vi "rec_manipMultiJumpDAQreplicates_v02.vi"(0 "AI task in":refnum<k21>, 1 "number of samples":i32=-1, 2 "Jump Position Array":T1(array[ring]), 3 "controls array in":refnum<vi>[](array[refnum]), 4 "AO task in":refnum<k21>, 5 "error in":errorcluster, 6 "Start Position":T2(ring), 7 "Delay":dbl, 8 "Use Current Position for Start Pos?":bool, 9 "Duration (s)":dbl, 11 "Position Dwell Time (s)":dbl[](array[numeric]), 12 "common cluster":T3) -> (14 "AI task out":refnum<k21>, 15 "data out (pA or mV)":waveform(dbl)(graph), 17 "control array out":refnum<vi>[](array[refnum]), 18 "AO task out":refnum<k21>, 19 "error out":errorcluster)   [LabVIEW 2019]
uses:
  multipatch/controls/multipatch_common_controls_v4.ctl
  machine_vision/controls/transform_cluster_actuator.ctl
  machine_vision/coordinate model vis/transform_properties_actuators.ctl
  pipette cleaning/pressure box/cleaning_soft/controls/actuator_cluster.ctl
  pipette cleaning/pressure box/cleaning_soft/controls/actuator_type.ctl
  pipette cleaning/pressure box/cleaning_soft/controls/pressure_box_control.ctl
  pipette cleaning/pressure box/cleaning_soft/controls/pressure_box_type.ctl
  controls/NH_method.ctl
  <vilib>/DAQmx/read.llb/DAQmx Read (Analog Wfm 1Chan NSamp).vi
  <vilib>/DAQmx/miscellaneous.llb/DAQmx Fill In Error Info.vi
  <resource>/objmgr/daqmx.rc
panel:
  out "AvailSampPerChan":u32
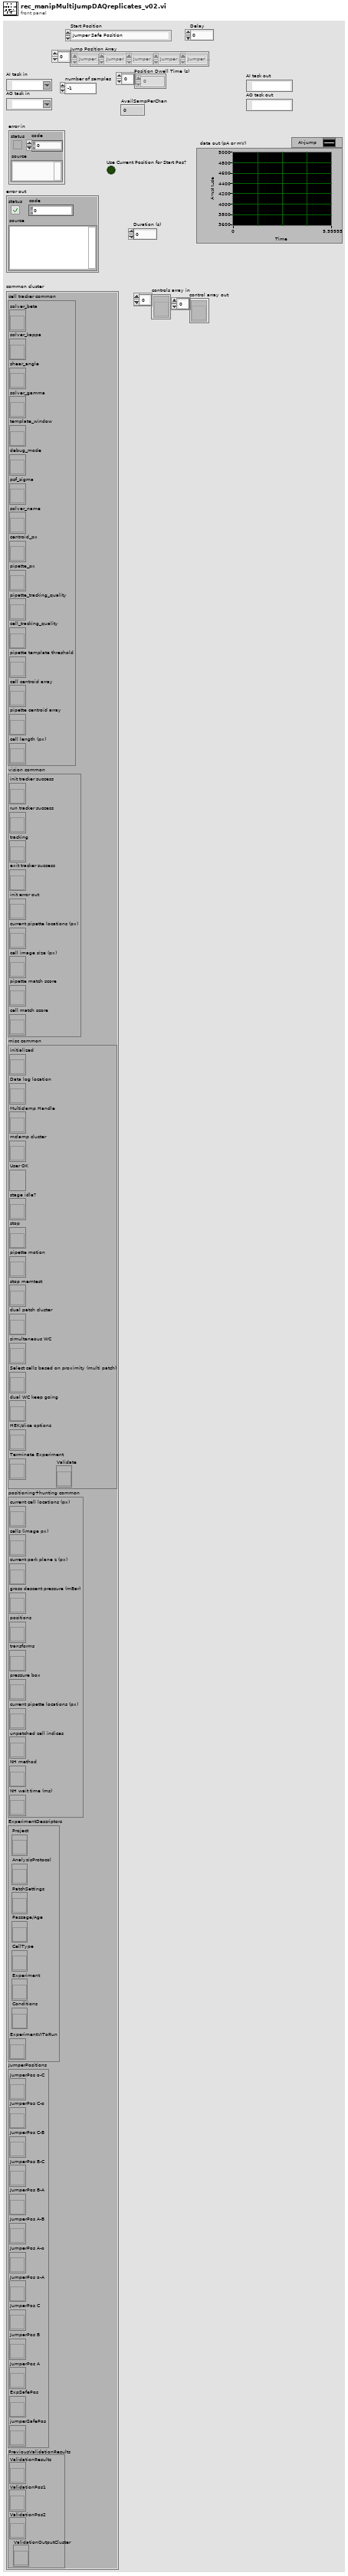
[diagram p1: front panel]
types:
  T1 = enum16{"Jumper Safe Position", "Experiment Safe Position", "Jumper Position A", "Jumper Position B", "Jumper Position C", "Jumper Position o-A", "Jumper Position A-o", "Jumper Position A-B", "Jumper Position B-A", "Jumper Position B-C", "Jumper Position C-B", "Jumper Position C-o", "Jumper Position o-C"}[]
  T2 = enum16{"Jumper Safe Position", "Experiment Safe Position", "Jumper Position A", "Jumper Position B", "Jumper Position C", "Jumper Position o-A", "Jumper Position A-o", "Jumper Position A-B", "Jumper Position B-A", "Jumper Position B-C", "Jumper Position C-B", "Jumper Position C-o", "Jumper Position o-C"}
  T3 = typedef "multipatch_common_controls_v4.ctl" = cluster{"cell tracker common":cluster{"solver_beta":refnum<vi>, "solver_kappa":refnum<vi>, "shear_angle":refnum<vi>, "solver_gamma":refnum<vi>, "template_window":refnum<vi>, "debug_mode":refnum<vi>, "psf_sigma":refnum<vi>, "solver_name":refnum<vi>, "centroid_px":refnum<vi>, "pipette_px":refnum<vi>, "pipette_tracking_quality":refnum<vi>, "cell_tracking_quality":refnum<vi>, "pipette template threshold":refnum<vi>, "cell centroid array":refnum<vi>, "pipette centroid array":refnum<vi>, "cell length (px)":refnum<vi>}, "vision common":cluster{"init tracker success":refnum<vi>, "run tracker success":refnum<vi>, "tracking":refnum<vi>, "exit tracker success":refnum<vi>, "init error out":refnum<vi>, "current pipette locations (px)":refnum<vi>, "cell image size (px)":refnum<vi>, "pipette match score":refnum<vi>, "cell match score":refnum<vi>}, "misc common":cluster{"initialized":refnum<vi>, "Data log location":refnum<vi>, "Multiclamp Handle":refnum<vi>, "mclamp cluster":refnum<vi>, "User OK":refnum<vi>, "stage idle?":refnum<vi>, "stop":refnum<vi>, "pipette motion":refnum<vi>, "stop memtest":refnum<vi>, "dual patch cluster":refnum<vi>, "simultaneous WC":refnum<vi>, "Select cells based on proximity (multi patch)":refnum<vi>, "dual WC keep going":refnum<vi>, "HEK/slice options":refnum<vi>, "Terminate Experiment":refnum<vi>, "Validate":refnum<vi>}, "positioning+hunting common":cluster{"current cell locations (px)":refnum<vi>, "cells (image px)":refnum<vi>, "current park plane z (px)":refnum<vi>, "gross descent pressure (mBar)":refnum<vi>, "positions":refnum<vi>, "transforms":refnum<vi>, "pressure box":refnum<vi>, "current pipette locations (px)":refnum<vi>, "unpatched cell indices":refnum<vi>, "NH method":refnum<vi>, "NH wait time (ms)":refnum<vi>}, "ExperimentDescriptors":cluster{"Project":refnum<vi>, "AnalysisProtocol":refnum<vi>, "PatchSettings":refnum<vi>, "Passage/Age":refnum<vi>, "CellType":refnum<vi>, "Experiment":refnum<vi>, "Conditions":refnum<vi>, "ExperimentVIToRun":refnum<vi>}, "JumperPositions":cluster{"JumperPos o-C":refnum<vi>, "JumperPos C-o":refnum<vi>, "JumperPos C-B":refnum<vi>, "JumperPos B-C":refnum<vi>, "JumperPos B-A":refnum<vi>, "JumperPos A-B":refnum<vi>, "JumperPos A-o":refnum<vi>, "JumperPos o-A":refnum<vi>, "JumperPos C":refnum<vi>, "JumperPos B":refnum<vi>, "JumperPos A":refnum<vi>, "ExpSafePos":refnum<vi>, "jumperSafePos":refnum<vi>}, "PreviousValidationResults":cluster{"ValidationResults":refnum<vi>, "ValidationPos1":refnum<vi>, "ValidationPos2":refnum<vi>, "ValidationOutputCluster":refnum<vi>}}
  T4 = enum16{"manipulator 1", "manipulator 2", "manipulator 3", "manipulator 4"}
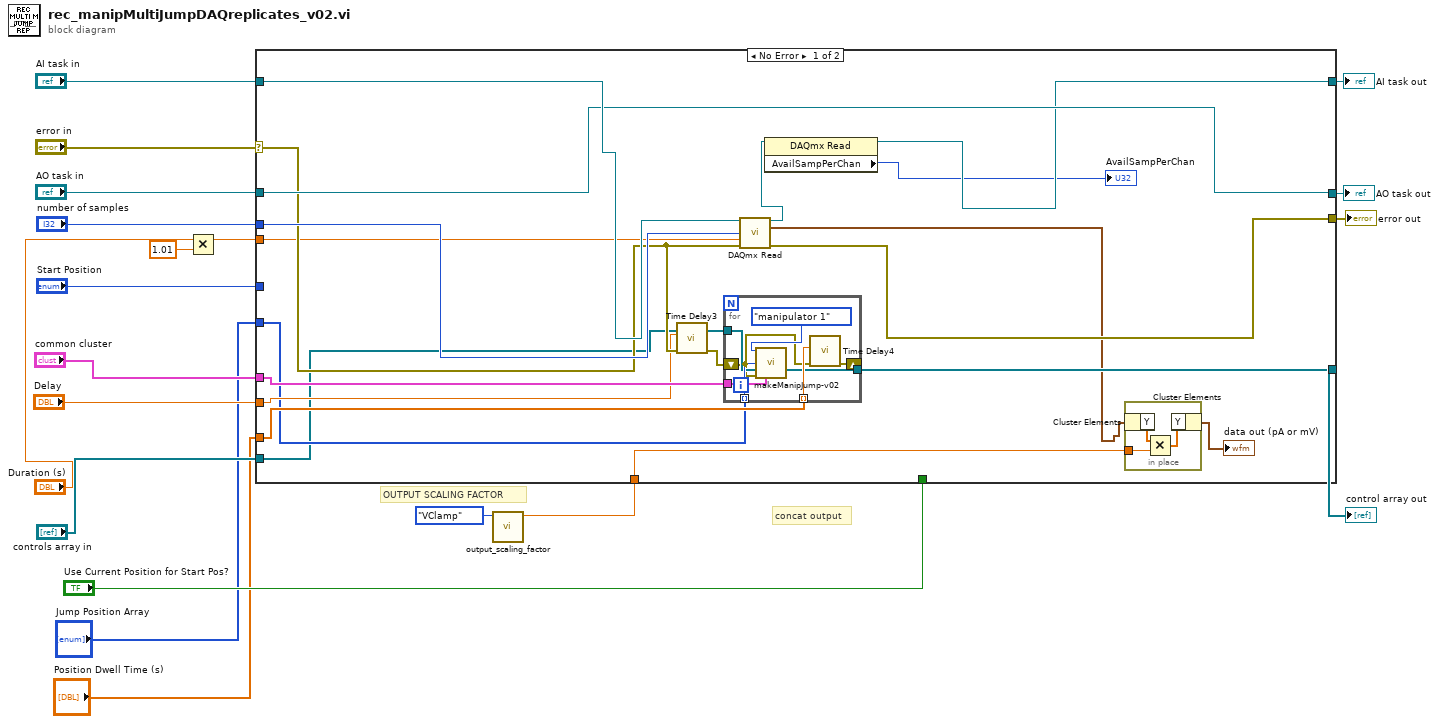
[diagram p0: block diagram]
diagram:
  # "concat output"
  # "OUTPUT SCALING FACTOR"
  n1 = Multiply(x="Duration (s)", y=1.01) -> (x*y=w5:dbl)
  n2 = call "output_scaling_factor.vi"("which clamp"=enum16{"VClamp", "IClamp"}."VClamp") -> ("output scaling factor"=w14:dbl)  [unwired: 10 in]
  n3 = case shown="No Error" "error in" {
    selector: "error in" -> [w34 w52]
    tunnel: "AI task in" -> [w38 w54]
    tunnel: "AO task in" -> [w36 w53]
    tunnel: [w36 w53] -> w17
    tunnel: [w27 w54] -> w16
    tunnel: [w37 w52] -> w15
    tunnel: w14 -> [w39 _]
    tunnel: "number of samples" -> [w35 _]
    tunnel: "common cluster" -> [w33 _]
    tunnel: "Delay" -> [w32 _]
    tunnel: "Position Dwell Time (s)" -> [w31 _]
    tunnel: "Start Position" -> [_ _]
    tunnel: "Jump Position Array" -> [w30 _]
    tunnel: "controls array in" -> [w29 w51]
    tunnel: [w28 w51] -> w7
    tunnel: w5 -> [w25 _]
    tunnel: "Use Current Position for Start Pos?" -> [_ _]
    frame No Error {
      n4 = call "Time Delay3"("error in (no error)"=w34, "Delay Time (s)"=w32) -> ("error out"=w23:errorcluster)  [unwired: 9 in]
      n5 = for {
        tunnel: w33 -> [w50]
        tunnel: w31 -> [w49] mode=indexing
        tunnel: w30 -> [w47] mode=indexing
        tunnel: w29 -> [w46]
        tunnel: [w45] -> w28
        shift-right: [w44] -> _
        shift-left: w23 -> [w43]
        n6 = call "makeManipJump-v02.vi"("which manipulator"=T4."manipulator 1", "Which Jumper Position to move to?"=w47, "controls array in"=w46, "error in"=w43, "common cluster"=w50) -> ("control array out"=w45:refnum<vi>[])  [unwired: 8 in, 2 out]
        n7 = call "Time Delay4"("error in (no error)"=w43, "Delay Time (s)"=w49) -> ("error out"=w44:errorcluster)  [unwired: 9 in]
      }
      n8 = call-poly <vilib>:"DAQmx Read.vi"("task/channels in"=w38, "number of samples per channel"=w35, "timeout"=w25, "error in"=w34) -> ("task out"=w24:refnum<k21>, "data"=w22:waveform(dbl), "error out"=w37:errorcluster)  [unwired: 9 in]
      n9 = property class="DAQmx Read"(reference=w24) -> (reference out=w27:refnum<k21>, "AvailSampPerChan"=→"AvailSampPerChan":u32)  [unwired: 1 in, 1 out]
      n10 = in-place {
        in-place-border: w39 -> [w42]
        n11 = in-place-cluster #1(w22) -> ("Y"=w41:dbl[])
        n12 = Multiply(x=w41, y=w42) -> (x*y=w40:dbl[])
        n13 = in-place-cluster #1("Y"=w40) -> (→"data out (pA or mV)":waveform(dbl))
      }
    }
    frame Error {
    }
  }
  "AI task out" <- w16
  "AO task out" <- w17
  "error out" <- w15
  "control array out" <- w7
